vi "Write Buffer to Log.vi"() -> ()   [LabVIEW 2018]
uses:
  Huskie Board.ctl
panel:
  out "error out":errorcluster
  in  "error in":errorcluster
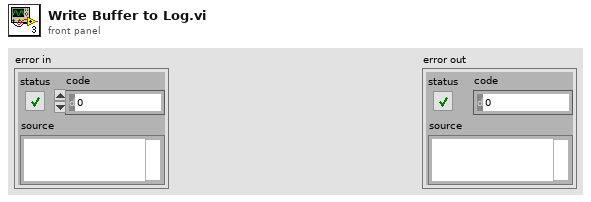
[diagram p1: front panel]
types:
  T1 = typedef "Huskie Board.ctl" = enum16{"Huskie Board", "Logging Queue"}
  T2 = typedef "WPI_SerialPortRef.ctl" = cluster{"DevStatus":errorcluster, "Serial Port Name":refnum<visa-resource-name>}
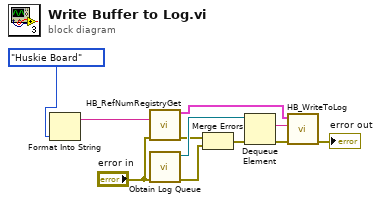
[diagram p0: block diagram]
diagram:
  n1 = Format Into String(Huskie_Board."Huskie Board" ("Enum")) -> (resulting string=w2:string)  [unwired: 3 in, 1 out]
  n2 = call <vilib>:"HB_RefNumRegistryGet.vi"("refnum name"=w2, "error in (no error)"="error in") -> ("HBDevRef"=w11:T2, "error out"=w6:errorcluster)  [unwired: 12 in]
  n3 = call "Obtain Log Queue.vi"("error in"="error in") -> ("error out"=w5:errorcluster, "queue out"=w9:refnum<queue>)  [unwired: 9 in]
  n4 = Merge Errors(w6, w5) -> (w7:errorcluster)
  n5 = Dequeue Element(queue=w9, error in (no error)=w7) -> (element=w8:string, error out=w4:errorcluster)  [unwired: 1 in, 2 out]
  n6 = call "HB_WriteToLog.vi"("error in (no error)"=w4, "Log string"=w8, "HBDevRef"=w11) -> ("error out"=→"error out":errorcluster)  [unwired: 7 in, 1 out]
